vi "ConvertSCPIValueToBoolean.vi"(11 "SCPI Value":string) -> (3 "Boolean":bool)   [LabVIEW 8.6, in "Keithley-6482-Visa.lvlib"]
uses:
  Keithley-6482-Visa.lvlib
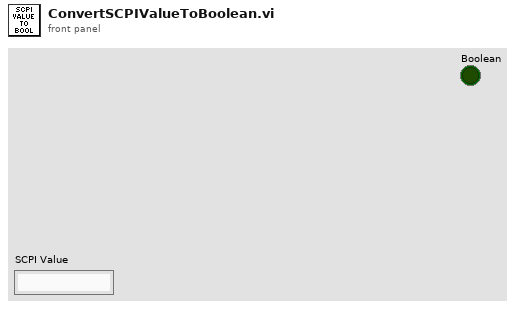
[diagram p1: front panel]
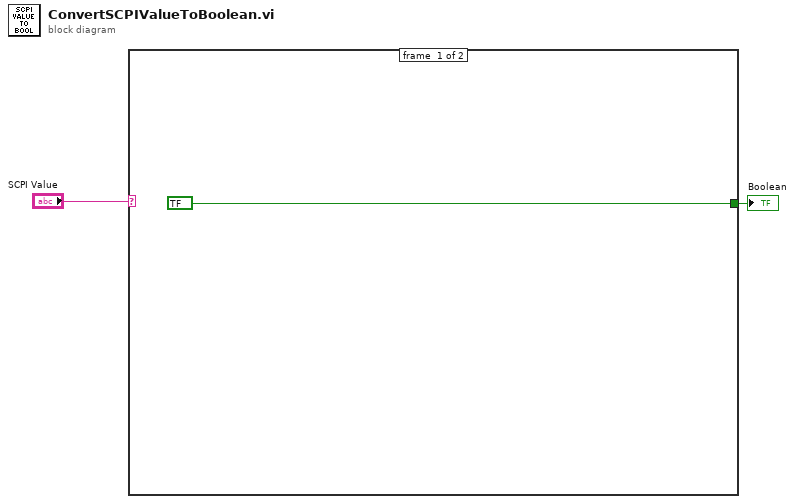
[diagram p0: block diagram]
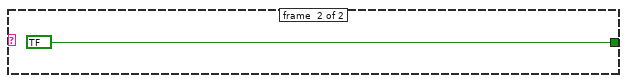
[diagram p2: hidden frame]
diagram:
  n1 = case shown="\"ON\"" "SCPI Value" {
    tunnel: [bool ? bool ?] -> w1
    frame #0 {
    }
    frame #1 {
    }
  }
  "Boolean" <- w1
